vi "TCP单点接收.main.vi"(0 "IP地址":string="127.0.0.1" caption="对方公网访问地址", 1 "端口号":i32=6314, 2 "储存路径":path=path "D:/AA", 3 "停止":bool, 5 "error IO":errorcluster caption="错误输入") -> (14 "已收百分比":string, 15 "运行指示灯":bool, 19 "错误输出 2":errorcluster caption="错误输出")   [LabVIEW 2016, in "数据传输系统-05.lvlib" / "自动更新.lvlib" / "TCP文件传输系统.lvlib" / "TCP接收文件.lvlib"]
panel:
  out "数值":i32
  in  "分一包（兆）":i64=40
  out "文件名":string
  out "2":errorcluster caption="错误输出"
  out "单包大小":i32
  out "帧数":i32
  out "帧号":i32
  out "错误输出":errorcluster
  out "路径 2":path
  out "已收次数":i32
  out "需接收次数":i32
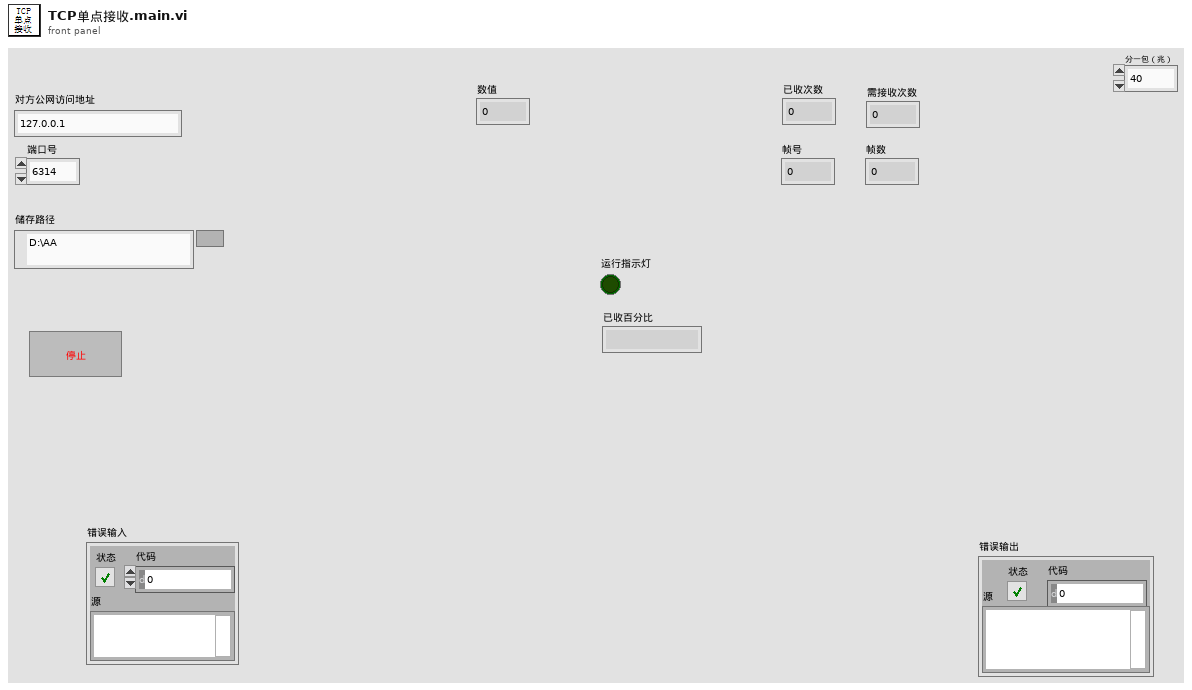
[diagram p1: front panel]
types:
  T1 = cluster{"网络灯":bool, "接收中":bool, "已接收百分比":u8, "接收成功次数":dbl, "当前步骤":enum16{"init", "receivehead", "receivecontent", "receivesuccess", "over"}, "文件名":string, "error out":errorcluster}
  T2 = enum16{"open", "replace", "create", "open or create", "replace or create", "replace or create with confirmation"}
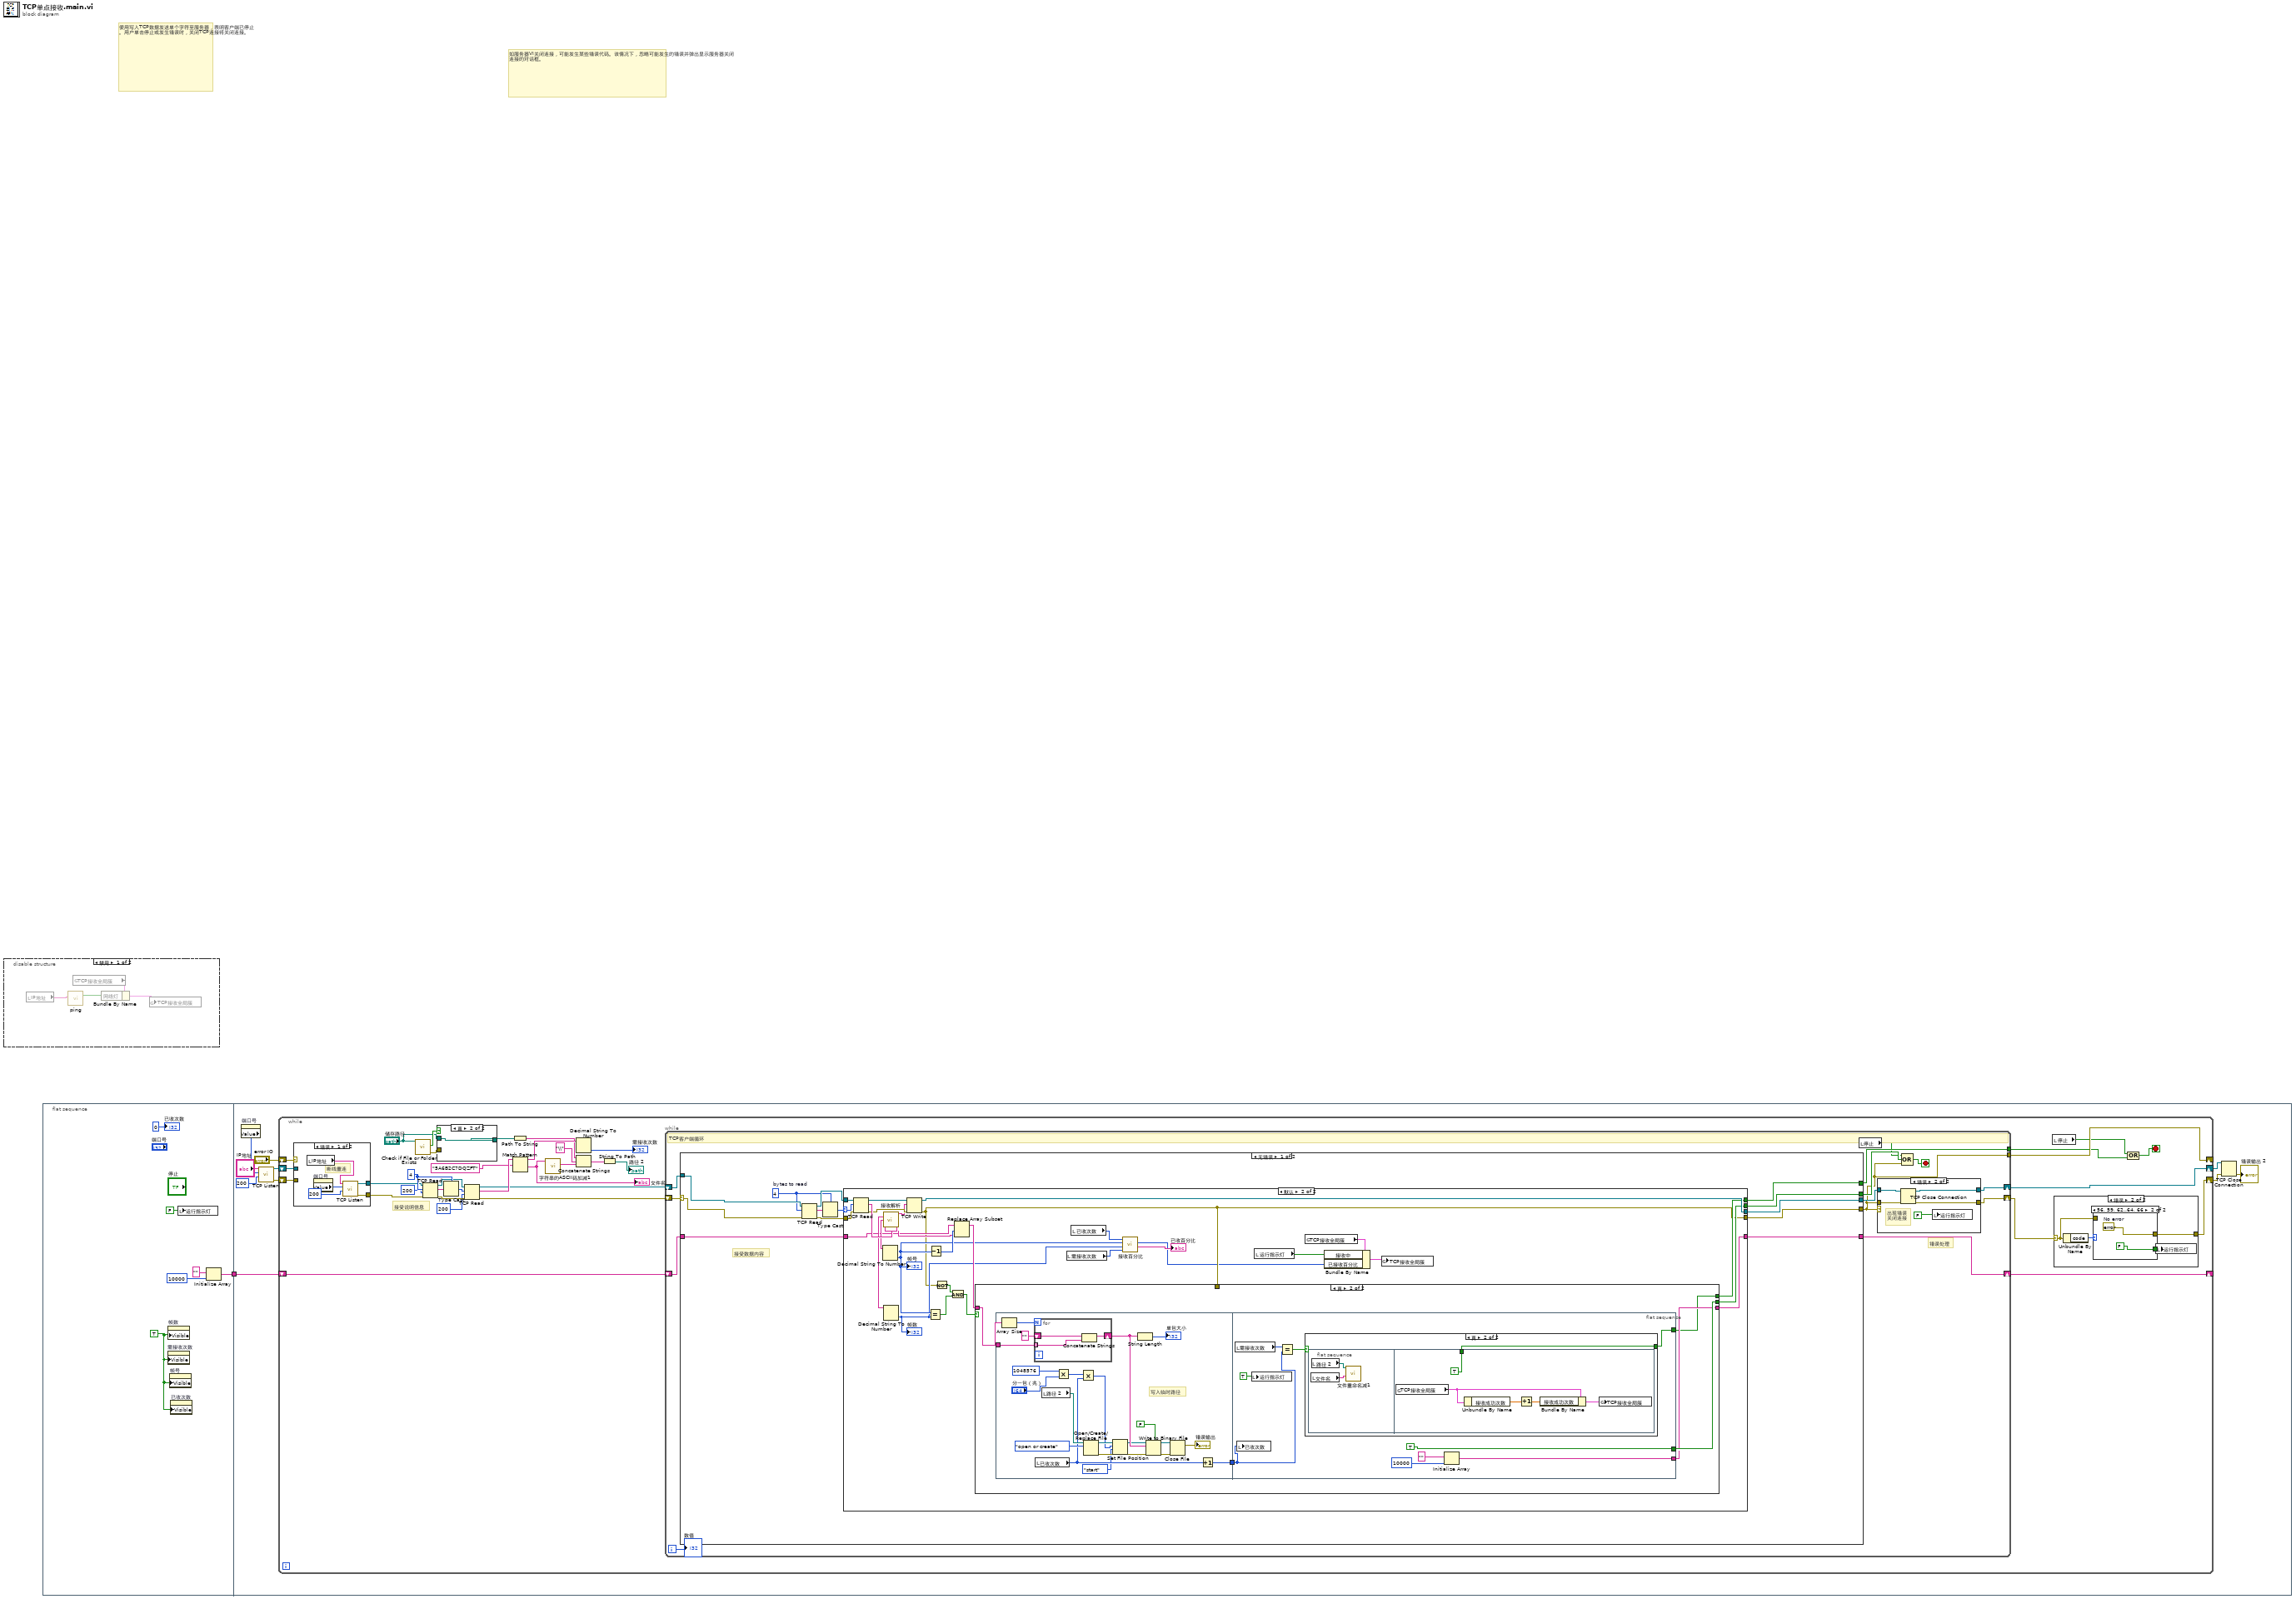
[diagram p0: block diagram]
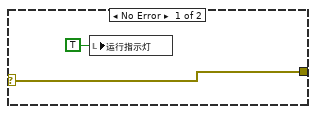
[diagram p3: hidden frame]
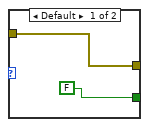
[diagram p4: hidden frame]
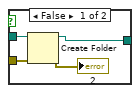
[diagram p5: hidden frame]
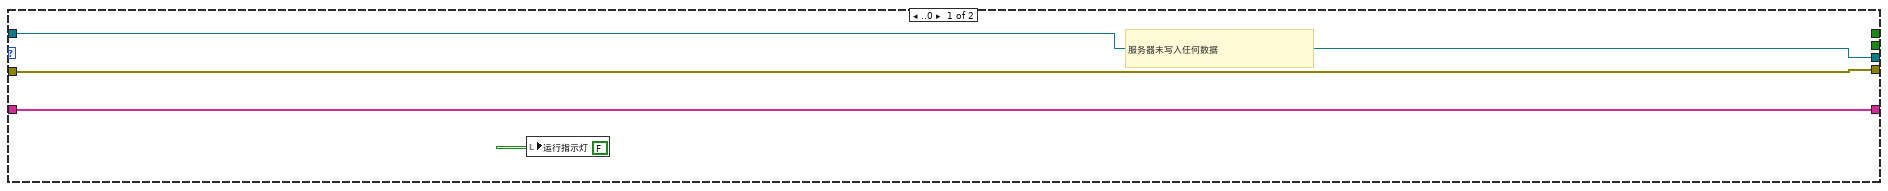
[diagram p8: hidden frame]
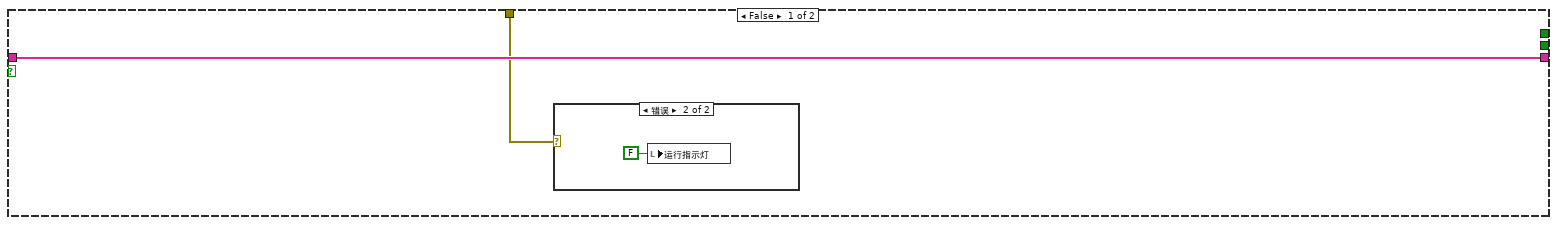
[diagram p9: hidden frame]
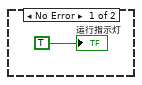
[diagram p10: hidden frame]
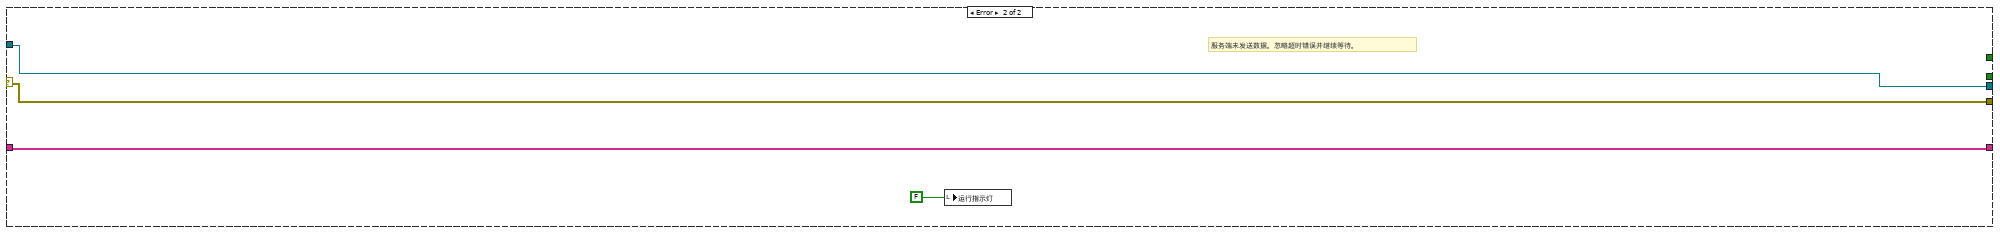
[diagram p12: hidden frame]
diagram:
  # "如服务器VI关闭连接，可能发生某些错误代码。该情况下，忽略可能发生的错误并弹出显示服务器关闭连接的对话框。"
  # "使用写入TCP数据发送单个字符至服务器，表明客户端已停止。用户单击停止或发生错误时，关闭TCP连接将关闭连接。"
  n1 = disable-structure shown="禁用" {
    frame Disabled {
      n2 = local read "IP地址"() -> (w5:string)
      n3 = call "ping.vi"("IP"=w5) -> ("ping结果"=w2:bool)  [unwired: 10 in]
      n4 = global read "全局变量1.vi" "TCP接收全局簇"() -> (w3:T1)
      n5 = Bundle By Name(cluster=w3, "网络灯"=w2) -> (w4:T1)
      n6 = global write "全局变量1.vi" "TCP接收全局簇"(w4) -> ()
    }
    frame Enabled {
    }
  }
  n7 = flat-sequence {
    tunnel: [w8] -> w1
    tunnel: w1 -> [w21]
    frame #0 {
      w7 = TRUE ("可见")
      n8 = property on="需接收次数" class="DigNum (严格)"("Visible"=w7) -> ()  [unwired: 2 in, 2 out]
      n9 = property on="帧数" class="DigNum (严格)"("Visible"=w7) -> ()  [unwired: 2 in, 2 out]
      n10 = property on="帧号" class="DigNum (严格)"("Visible"=w7) -> ()  [unwired: 2 in, 2 out]
      n11 = property on="已收次数" class="DigNum (严格)"("Visible"=w7) -> ()  [unwired: 2 in, 2 out]
      n12 = local write "运行指示灯"(FALSE ("运行指示灯")) -> ()
      n13 = Initialize Array("", 10000 ("维数大小")) -> (w8:string[])
      "已收次数" <- i64 0 ("已发次数")
    }
    frame #1 {
      n14 = property on="端口号" class="DigNum (严格)"() -> ("Value"=w15:i32)  [unwired: 2 in, 2 out]
      n15 = call <vilib>:"TCP Listen.vi"("timeout ms (wait forever: -1)"=200, "port"=w15, "service name"="IP地址") -> ("error out"=w20:errorcluster, "connection ID"=w19:refnum<k5>)  [unwired: 4 in, 3 out]
      n16 = while {
        shift-right: [w44] -> _
        shift-left: w21 -> [w43]
        shift-right: [w58] -> w17
        shift-left: w19 -> [w42]
        shift-right: [w28] -> w18
        shift-left: w20 -> [w41]
        shift-right: [w39] -> _
        shift-left: "error IO" -> [w38]
        stop <- w22 stop-if-true
        w57 = 4 ("读取的字节")
        # "接受说明信息"
        n17 = case shown="错误" w38 {
          tunnel: w42 -> [_ w80]
          tunnel: [w78 w80] -> w27
          tunnel: w41 -> [_ w79]
          tunnel: [w77 w79] -> w26
          frame Error {
            # "断线重连"
            n18 = local read "IP地址"() -> (w75:string)
            n19 = property on="端口号" class="DigNum (严格)"() -> ("Value"=w76:i32)  [unwired: 2 in, 2 out]
            n20 = call <vilib>:"TCP Listen.vi"("timeout ms (wait forever: -1)"=200, "port"=w76, "service name"=w75) -> ("error out"=w77:errorcluster, "connection ID"=w78:refnum<k5>)  [unwired: 4 in, 3 out]
          }
          frame No Error {
          }
        }
        n21 = call <vilib>:"Check if File or Folder Exists.vi"("path"="储存路径") -> ("error out"=w36:errorcluster, "file or folder exists?"=w37:bool)  [unwired: 8 in, 1 out]
        n22 = TCP Read(connection ID=w27, bytes to read=w57, error in (no error)=w26, 9:200 ("超时毫秒(25000)")) -> (connection ID out=w53:refnum<k5>, data out=w56:string, error out=w54:errorcluster)  [unwired: 1 in]
        n23 = case shown="真" w37 {
          tunnel: "储存路径" -> [w72 w73]
          tunnel: w36 -> [w71 _]
          tunnel: [w70 w73] -> w33
          frame False {
            n24 = Create Folder(path (use dialog)=w72, error in=w71) -> (created path=w70:path, error out=→"2":errorcluster)  [unwired: 1 in, 1 out]
          }
          frame True {
          }
        }
        n25 = Type Cast(type=w57, x=w56) -> (*(type *) &x=w55:i32)
        n26 = TCP Read(connection ID=w53, bytes to read=w55, error in (no error)=w54, 9:200 ("超时毫秒(25000)")) -> (connection ID out=w40:refnum<k5>, data out=w52:string, error out=w30:errorcluster)  [unwired: 1 in]
        n27 = Path To String(path=w33) -> (string=w34:string)
        n28 = Match Pattern(string=w52, regular expression="5A6B2C7DQZFT" ("正则表达式")) -> (before substring=w50:string, after substring=w32:string)  [unwired: 1 in, 2 out]
        "文件名" <- w32
        n29 = call "字符串的ASCII码加减1.vi"("原字符串"=w32) -> ("ASCII码"=w31:string)  [unwired: 10 in]
        n30 = Decimal String To Number(string=w50) -> (number=→"需接收次数":i32)  [unwired: 2 in, 1 out]
        n31 = Concatenate Strings(w34, "\\" ("字符串"), w31) -> (w48:string)
        n32 = String To Path(string=w48) -> (path=→"路径 2":path)
        n33 = while {
          tunnel: [w90] -> w23
          shift-right: [w89] -> w44
          shift-left: w43 -> [w88]
          shift-right: [w83] -> w29
          shift-left: w30 -> [w92]
          shift-right: [w86] -> w58
          shift-left: w40 -> [w85]
          tunnel: [w84] -> w39
          i -> [w81]
          stop <- w93 stop-if-true
          # "错误处理"
          # "TCP客户端循环"
          n34 = case shown="无错误" w92 {
            selector: w92 -> [w112 w199]
            tunnel: [w111 w199] -> w84
            tunnel: w85 -> [w113 w200]
            tunnel: [w110 w200] -> w87
            tunnel: [w109 _] -> w91
            tunnel: [w108 _] -> w90
            tunnel: [w107 w202] -> w89
            tunnel: w88 -> [w106 w202]
            frame No Error {
              w103 = 4  # bytes to read
              # "接受数据内容"
              n35 = TCP Read(connection ID=w113, bytes to read=w103, error in (no error)=w112) -> (connection ID out=w105:refnum<k5>, data out=w101:string, error out=w104:errorcluster)  [unwired: 2 in]
              n36 = Type Cast(type=w103, x=w101) -> (*(type *) &x=w102:i32)
              n37 = case shown="默认" w102 {
                selector: w102 -> [_ w145]
                tunnel: w105 -> [w117 w147]
                tunnel: w104 -> [w116 w146]
                tunnel: [w117 w139] -> w110
                tunnel: [w116 w123] -> w111
                tunnel: [_ w137] -> w109
                tunnel: [_ w134] -> w108
                tunnel: [w115 w131] -> w107
                tunnel: w106 -> [w115 w132]
                frame ..0 {
                  # "服务器未写入任何数据"
                  n38 = local write "运行指示灯"(FALSE ("运行指示灯")) -> ()
                }
                frame Default {
                  n39 = TCP Read(connection ID=w147, bytes to read=w145, error in (no error)=w146) -> (connection ID out=w141:refnum<k5>, data out=w144:string, error out=w140:errorcluster)  [unwired: 2 in]
                  n40 = call "接收解析.vi"("data in"=w144) -> ("重算CRC32"=w136:string, "帧数"=w138:string, "帧号"=w143:string, "帧内容"=w135:string)  [unwired: 3 in, 8 out]
                  n41 = Decimal String To Number(string=w143) -> (number=w128:i32)  [unwired: 2 in, 1 out]
                  "帧号" <- w128
                  n42 = Decimal String To Number(string=w138) -> (number=w127:i32)  [unwired: 2 in, 1 out]
                  "帧数" <- w127
                  n43 = TCP Write(connection ID=w141, data in=w136, error in (no error)=w140) -> (connection ID out=w139:refnum<k5>, error out=w123:errorcluster)  [unwired: 1 in, 1 out]
                  n44 = Equal?(x=w128, y=w127) -> (x = y?=w126:bool)
                  n45 = Decrement(x=w128) -> (x-1=w142:i32)
                  n46 = Not(x=w123) -> (.not. x?=w125:bool)
                  n47 = And(x=w125, y=w126) -> (x .and. y?=w124:bool)
                  n48 = Replace Array Subset(array=w132, new element=w135, index=w142) -> (w133:string[])
                  n49 = case shown="真" w124 {
                    tunnel: [_ w155] -> w137
                    tunnel: w133 -> [w149 w156]
                    tunnel: [_ w152] -> w134
                    tunnel: [w149 w153] -> w131
                    tunnel: w123 -> [w148 _]
                    frame False {
                      n50 = case shown="错误" w148 {
                        frame No Error {
                          "运行指示灯" <- TRUE ("运行指示灯")
                        }
                        frame Error {
                          n51 = local write "运行指示灯"(FALSE ("运行指示灯")) -> ()
                        }
                      }
                    }
                    frame True {
                      n52 = flat-sequence {
                        tunnel: w156 -> [w169]
                        tunnel: [w177] -> w154
                        tunnel: [TRUE] -> w155
                        tunnel: w154 -> [w189]
                        tunnel: [w186] -> w152
                        tunnel: [w183] -> w153
                        frame #0 {
                          # "写入临时路径"
                          n53 = Array Size(array=w169) -> (size(s)=w170:i32)
                          n54 = for {
                            N: w170 -> [_]
                            shift-right: [w181] -> w168
                            shift-left: "" -> [w180]
                            tunnel: w169 -> [w179] mode=indexing
                            n55 = Concatenate Strings(w180, w179) -> (w181:string)
                          }
                          n56 = local read "已收次数"() -> (w162:i32)
                          n57 = local read "路径 2"() -> (w178:path)
                          n58 = Multiply(x=i64 1048576, y="分一包（兆）") -> (x*y=w158:i64)
                          n59 = Multiply(x=w158, y=w162) -> (x*y=w161:i64)
                          n60 = Open/Create/Replace File(file path (use dialog)=w178, operation (0:open)=T2."open or create" ("操作(0:open)")) -> (refnum out=w165:refnum<file>, error out=w166:errorcluster)  [unwired: 4 in, 1 out]
                          n61 = Set File Position(offset (in bytes) (0)=w161, refnum=w165, from (0:start)=enum16{"start", "end", "current"}."start" ("自（0:起始）"), error in=w166) -> (refnum out=w163:refnum<file>, error out=w164:errorcluster)
                          n62 = String Length(string=w168) -> (length=→"单包大小":i32)
                          n63 = Write to Binary File(file (use dialog)=w163, data=w168, error in=w164, 5:FALSE ("预置数组或字符串大小？(T)")) -> (refnum out=w175:refnum<file>, error out=w176:errorcluster)  [unwired: 2 in, 1 out]
                          n64 = Close File(refnum=w175, error in=w176) -> (error out=→"错误输出":errorcluster)  [unwired: 1 out]
                          n65 = Increment(x=w162) -> (x+1=w177:i32)
                        }
                        frame #1 {
                          n66 = local read "需接收次数"() -> (w188:i32)
                          n67 = local write "已收次数"(w189) -> ()
                          n68 = local write "运行指示灯"(TRUE ("运行指示灯")) -> ()
                          n69 = Equal?(x=w188, y=w189) -> (x = y?=w187:bool)
                          n70 = case shown="真" w187 {
                            tunnel: [_ w191] -> w186
                            frame False {
                            }
                            frame True {
                              n71 = flat-sequence {
                                tunnel: [TRUE] -> w191
                                frame #0 {
                                n72 = local read "文件名"() -> (w192:string)
                                n73 = local read "路径 2"() -> (w193:path)
                                n74 = call "文件重命名减1.vi"("名称或相对路径"=w192, "源路径"=w193) -> ()  [unwired: 10 in]
                                }
                                frame #1 {
                                n75 = global read "全局变量1.vi" "TCP接收全局簇"() -> (w194:T1)
                                n76 = Unbundle By Name(w194) -> ("接收成功次数"=w195:dbl)
                                n77 = Increment(x=w195) -> (x+1=w196:dbl)
                                n78 = Bundle By Name(cluster=w194, "接收成功次数"=w196) -> (w197:T1)
                                n79 = global write "全局变量1.vi" "TCP接收全局簇"(w197) -> ()
                                }
                              }
                            }
                          }
                          n80 = Initialize Array("", 10000 ("维数大小")) -> (w183:string[])
                        }
                      }
                    }
                  }
                  n81 = local read "需接收次数"() -> (w129:i32)
                  n82 = local read "已收次数"() -> (w130:i32)
                  n83 = call "接收百分比.vi"("需发送次数"=w129, "帧数"=w127, "帧号"=w128, "已收次数"=w130) -> (1:"已收百分比"=→"已收百分比":string, 2:"已收百分比"=w118:u8)  [unwired: 6 in]
                  n84 = local read "运行指示灯"() -> (w119:bool)
                  n85 = global read "全局变量1.vi" "TCP接收全局簇"() -> (w121:T1)
                  n86 = Bundle By Name(cluster=w121, "接收中"=w119, "已接收百分比"=w118) -> (w122:T1)
                  n87 = global write "全局变量1.vi" "TCP接收全局簇"(w122) -> ()
                }
              }
            }
            frame Error {
              # "服务端未发送数据。忽略超时错误并继续等待。"
              n88 = local write "运行指示灯"(FALSE ("运行指示灯")) -> ()
            }
          }
          n89 = local read "停止"() -> (w82:bool)
          n90 = case shown="错误" w84 {
            tunnel: [w95 w98] -> w83
            tunnel: w84 -> [w95 w99]
            tunnel: [w94 w97] -> w86
            tunnel: w87 -> [w94 w100]
            frame No Error {
            }
            frame Error {
              # "出现错误\n关闭连接"
              n91 = TCP Close Connection(connection ID=w100, error in (no error)=w99) -> (connection ID out=w97:refnum<k5>, error out=w98:errorcluster)  [unwired: 1 in]
              n92 = local write "运行指示灯"(FALSE ("运行指示灯")) -> ()
            }
          }
          n93 = Compound Arithmetic op=OR(w82, w91, w84) -> (w93:bool)
          "数值" <- w81
        }
        n94 = local read "停止"() -> (w24:bool)
        n95 = case shown="错误" w29 {
          selector: w29 -> [w60 w63]
          tunnel: [w60 w62] -> w28
          frame No Error {
            n96 = local write "运行指示灯"(TRUE ("运行指示灯")) -> ()
          }
          frame Error {
            n97 = Unbundle By Name(w63) -> ("code"=w64:i32)
            n98 = case shown="56, 59, 62..64, 66" w64 {
              tunnel: w63 -> [w66 _]
              tunnel: [w66 w68] -> w62
              tunnel: [FALSE FALSE] -> w61
              frame Default {
              }
              frame 56, 59, 62..64, 66 {
                w68 = errorcluster {"status"=FALSE, "code"=0, "source"=""}  # No error
              }
            }
            n99 = local write "运行指示灯"(w61) -> ()
          }
        }
        n100 = Compound Arithmetic op=OR(w24, w23) -> (w22:bool)
      }
      n101 = TCP Close Connection(connection ID=w17, error in (no error)=w18) -> (error out=→"错误输出 2":errorcluster)  [unwired: 1 in, 1 out]
    }
  }
